vi "Exercicio1110.vi"() -> ()   [LabVIEW 2017]
panel:
  out "Mensagem":string
  in  "?":bool
  out "Temperatura => 70ºC":bool
  out "30ºC =< Temperatura < 70ºC":bool
  out "Temperatura < 30ºC":bool
  out "Fahrenheit":dbl
  out "?":dbl(knob) scale=32.0..212.0
  out "Fahrenheit":dbl(slide) scale=0.0..212.0
  in  "Celsius":dbl(slide) scale=0.0..100.0
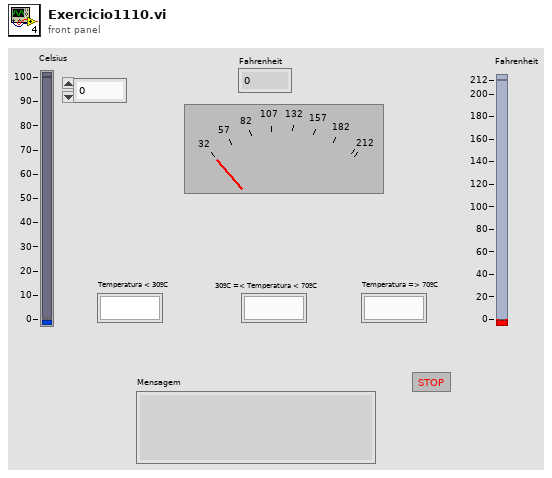
[diagram p1: front panel]
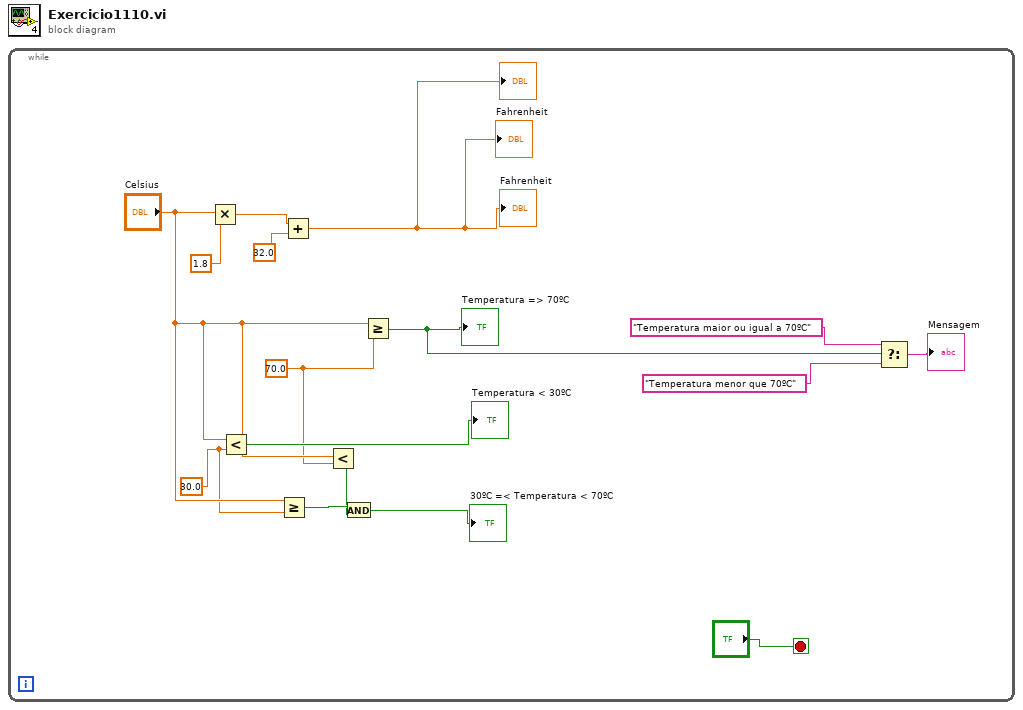
[diagram p0: block diagram]
diagram:
  n1 = while {
    stop <- "?" stop-if-true
    w5 = 30.0
    w8 = 70.0
    n2 = Multiply(x="Celsius", y=1.8) -> (x*y=w15:dbl)
    n3 = Less?(x="Celsius", y=w5) -> (x < y?=→"Temperatura < 30ºC":bool)
    n4 = Greater Or Equal?(x="Celsius", y=w5) -> (x >= y?=w10:bool)
    n5 = Add(x=w15, y=32.0) -> (x+y=→"Fahrenheit" →"?" →"Fahrenheit":dbl)
    n6 = Less?(x="Celsius", y=w8) -> (x < y?=w7:bool)
    n7 = And(x=w10, y=w7) -> (x .and. y?=→"30ºC =< Temperatura < 70ºC":bool)
    n8 = Greater Or Equal?(x="Celsius", y=w8) -> (x >= y?=w2:bool)
    "Temperatura => 70ºC" <- w2
    n9 = Select(t="Temperatura maior ou igual a 70ºC", s=w2, f="Temperatura menor que 70ºC") -> (s? t:f=→"Mensagem":string)
  }
